vi "Asset Utilization Example.vi"() -> ()   [LabVIEW 2019]
uses:
  <vilib>/Skyline/Configuration/Configuration HTTP_class/NI Skyline Configuration HTTP.lvclass/NI Skyline Configuration HTTP.ctl
  <vilib>/Skyline/Configuration/Configuration HTTP_class/Open Configuration HTTP.vi
  <vilib>/Skyline/Configuration/HTTP/Open Configuration (Desktop).vi
  <vilib>/Skyline/Configuration/Configuration HTTP_class/NI Skyline Configuration HTTP.lvclass
  <vilib>/Skyline/Configuration/Configuration_class/NI Skyline Configuration.lvclass
panel:
  in  "Password":string
  in  "Username":string="admin"
  in  "Server":string="https://localhost"
  out "Past Asset Utilization":string[][](table)
  out "Assets In Use":string[][](table)
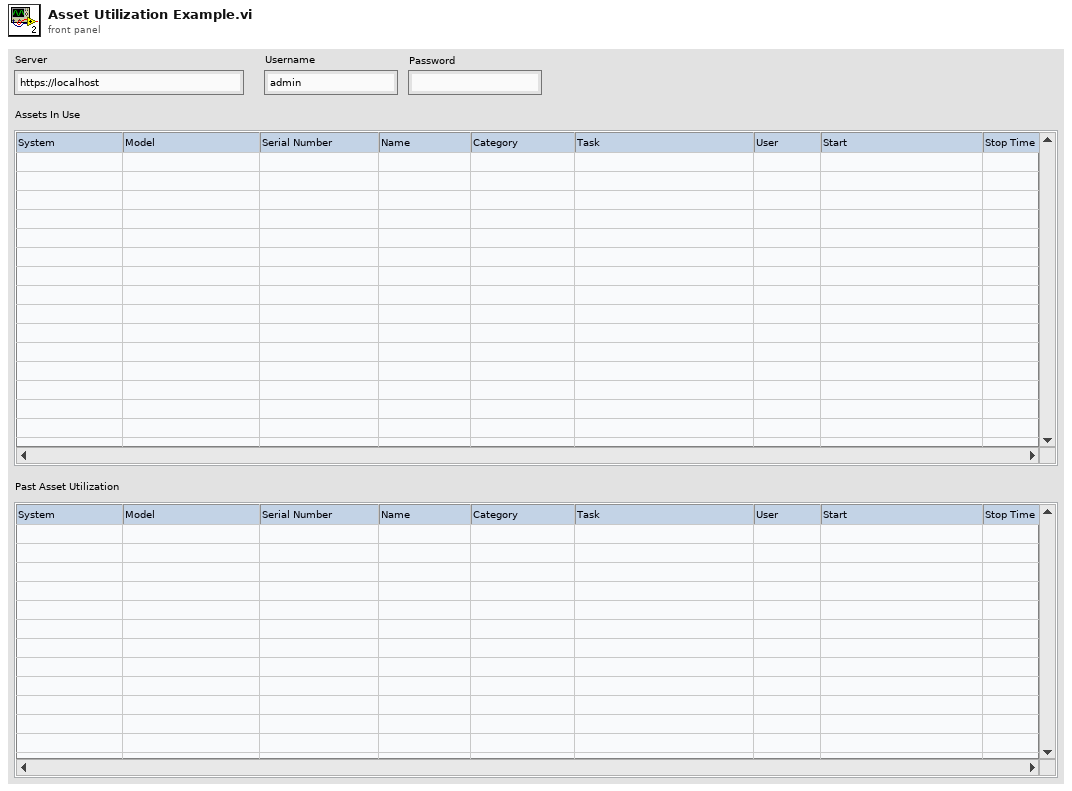
[diagram p1: front panel]
types:
  T1 = cluster{"utilizationIdentifier":string, "assetIdentifier":string, "minionId":string, "category":string, "taskName":string, "userName":string, "startTimestamp":string, "endTimestamp":string, "heartbeatTimestamp":string}[]
  T2 = cluster{"modelName":string, "serialNumber":string, "vendorName":string, "name":string, "location":cluster{"systemName":string}}
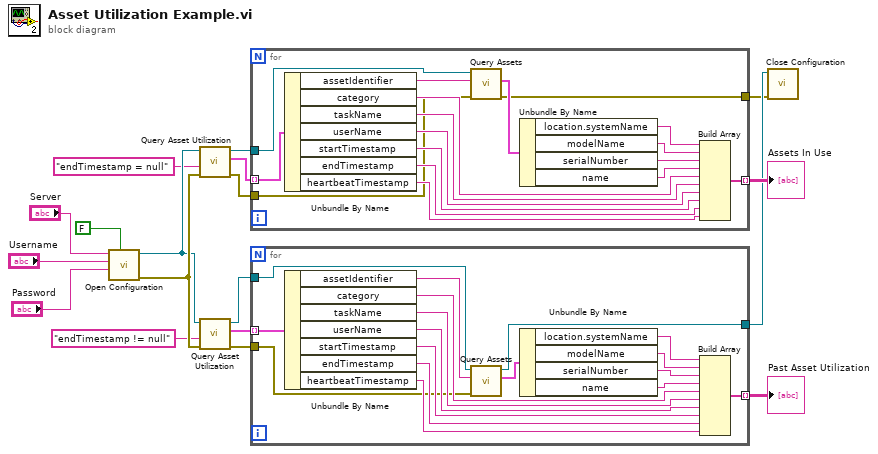
[diagram p0: block diagram]
diagram:
  n1 = call-poly <vilib>:"Open Configuration.vi"("verify server?"=FALSE, "password"="Password", "username"="Username", "server url"="Server") -> ("error out"=w10:errorcluster, "configuration"=w9:refnum<class "NI Skyline Configuration HTTP.lvclass">)  [unwired: 6 in]
  n2 = call "Query Asset Utilization.vi"("Error In"=w10, "Utilization Filter"="endTimestamp = null", "Session In"=w9) -> ("Error Out"=w14:errorcluster, "Asset Utilization"=w18:T1, "Session Out"=w15:refnum<class "NI Skyline Configuration HTTP.lvclass">)  [unwired: 6 in]
  n3 = call "Query Asset Utilization.vi"("Error In"=w10, "Utilization Filter"="endTimestamp != null" ("Asset Filter"), "Session In"=w9) -> ("Error Out"=w11:errorcluster, "Asset Utilization"=w13:T1, "Session Out"=w12:refnum<class "NI Skyline Configuration HTTP.lvclass">)  [unwired: 6 in]
  n4 = for {
    tunnel: w18 -> [w35] mode=indexing
    tunnel: [w28] -> w17 mode=indexing
    tunnel: w15 -> [w27]
    tunnel: w14 -> [w26]
    tunnel: [w19] -> w1
    n5 = Unbundle By Name(w35) -> ("assetIdentifier"=w20:string, "category"=w34:string, "taskName"=w33:string, "userName"=w32:string, "startTimestamp"=w31:string, "endTimestamp"=w30:string, "heartbeatTimestamp"=w29:string)
    n6 = call "Query Assets.vi"("Error In"=w26, "Asset ID"=w20, "Session In"=w27) -> ("Error Out"=w19:errorcluster, "Asset"=w21:T2)  [unwired: 6 in, 1 out]
    n7 = Unbundle By Name(w21) -> ("location.systemName"=w25:string, "modelName"=w24:string, "serialNumber"=w23:string, "name"=w22:string)
    n8 = Build Array(w25, w24, w23, w22, w34, w33, w32, w31, w30, w29) -> (w28:string[])
  }
  "Assets In Use" <- w17
  n9 = for {
    tunnel: w13 -> [w52] mode=indexing
    tunnel: [w45] -> w8 mode=indexing
    tunnel: w12 -> [w44]
    tunnel: w11 -> [w43]
    tunnel: [w36] -> w2
    n10 = Unbundle By Name(w52) -> ("assetIdentifier"=w37:string, "category"=w51:string, "taskName"=w50:string, "userName"=w49:string, "startTimestamp"=w48:string, "endTimestamp"=w47:string, "heartbeatTimestamp"=w46:string)
    n11 = call "Query Assets.vi"("Error In"=w43, "Asset ID"=w37, "Session In"=w44) -> ("Asset"=w38:T2, "Session Out"=w36:refnum<class "NI Skyline Configuration HTTP.lvclass">)  [unwired: 6 in, 1 out]
    n12 = Unbundle By Name(w38) -> ("location.systemName"=w42:string, "modelName"=w41:string, "serialNumber"=w40:string, "name"=w39:string)
    n13 = Build Array(w42, w41, w40, w39, w51, w50, w49, w48, w47, w46) -> (w45:string[])
  }
  "Past Asset Utilization" <- w8
  n14 = call-dynamic "Close Configuration.vi"("error in (no error)"=w1, "configuration"=w2) -> ()  [unwired: 9 in, 1 out]
